vi "TestTime_PublishAndObserve_OneTopic.vi"(8 "error in (no error)":errorcluster, 11 "TestCase in":refnum<class "BenchmarkObservationRate.lvclass">) -> (0 "error out":errorcluster, 3 "TestCase out":refnum<class "BenchmarkObservationRate.lvclass">)   [LabVIEW 2020, in "BenchmarkObservationRate.lvlib" / "BenchmarkObservationRate.lvclass"]
uses:
  BenchmarkObservationRate.lvclass
  BenchmarkObservationRate.lvclass/BenchmarkObservationRate.ctl
  24bf8875-c008-4f22-9bfa-88e42476d167.vi
  Source/IModel/IModel/IModel.lvclass
  <vilib>/ActorFramework/Actor/Actor.lvclass
  Source/Mediator/Mediator/Mediator.lvclass
  <vilib>/ActorFramework/Stop Msg/Stop Msg.lvclass
  Doubles/RootModelPublishesUnthrottled/ModelPublishesIndexA.lvclass
  Doubles/ModelCountsObservations/ModelTimesNObservations.lvclass
  Source/RootModel/RootModel/RootModel.lvclass
  C:/Git/mva-core/Source/IModel/IModel/IModel.lvclass
  C:/Git/mva-core/Source/IObserver/IObserver/IObserver.lvclass
  C:/Program Files (x86)/National Instruments/LabVIEW 2020/vi.lib/ActorFramework/Actor/Actor.lvclass
  C:/Git/mva-core/Source/RootModel/RootModel/RootModel.lvclass
  C:/Git/mva-core/Test/BechmarkObservationRate/Doubles/RootModelPublishesUnthrottled/ModelPublishesIndexA.lvclass
  C:/Git/mva-core/Test/BechmarkObservationRate/Doubles/ModelCountsObservations/ModelTimesNObservations.lvclass
panel:
  out "Publish-Observe Rate [Hz]":dbl
  out "Total Time [s]":dbl
  # "About 12 kHz typical in LV 2017"
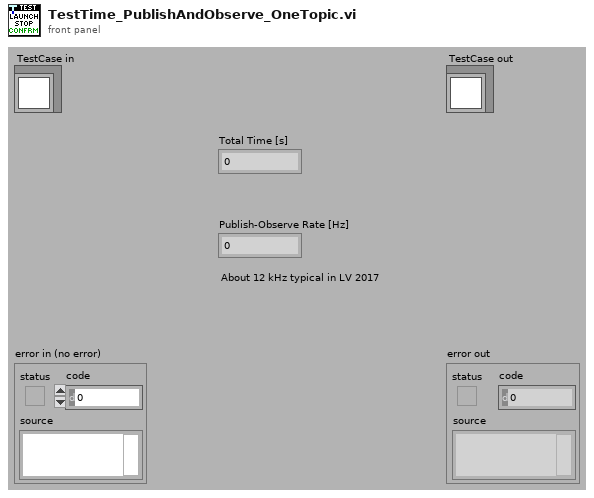
[diagram p1: front panel]
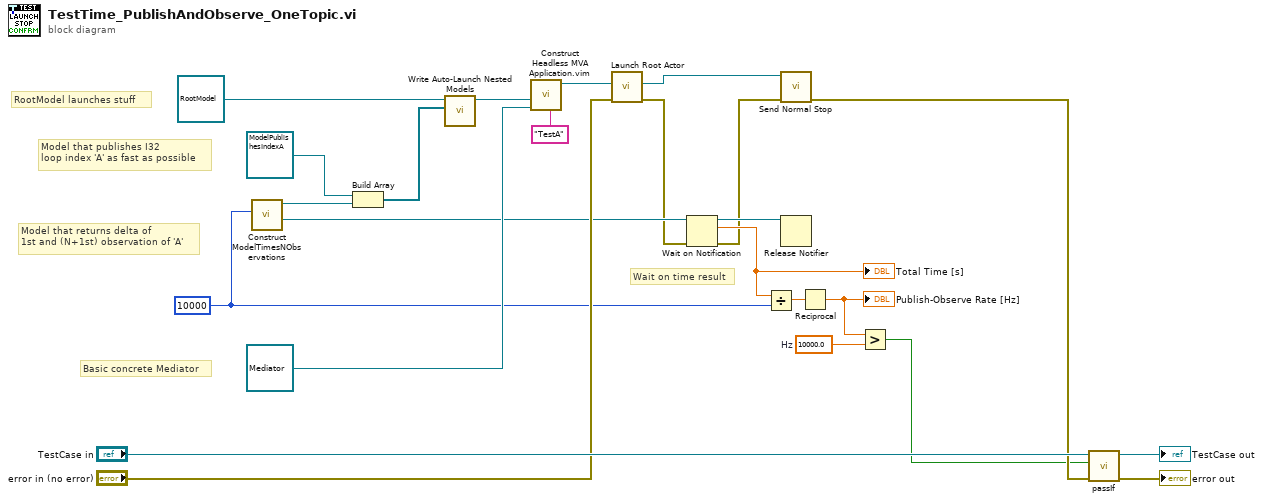
[diagram p0: block diagram]
diagram:
  w3 = 10000.0  # Hz
  w6 = 10000 ("Stop After N Observations")
  # "Wait on time result"
  # "RootModel launches stuff"
  # "Model that returns delta of\n1st and (N+1st) observation of 'A'"
  # "Model that publishes I32\nloop index 'A' as fast as possible"
  # "Basic concrete Mediator"
  n1 = call "Construct ModelTimesNObservations.vi"("Stop After N Observations"=w6) -> ("Elaped Seconds"=w13:refnum<notifier>, "ModelCountsObservations Out"=w12:refnum<class "ModelTimesNObservations.lvclass">)  [unwired: 9 in]
  n2 = Build Array(refnum<class "ModelPublishesIndexA.lvclass"> refnum ("BenchmarkObservationRate.lvlib:RootModelPublishesUnthrottled.lvclass"), w12) -> (w21:refnum<class "IModel.lvclass">[])
  n3 = call "Write Auto-Launch Nested Models.vi"("Auto-Launch Nested Models"=w21, "IModel In"=refnum<class "RootModel.lvclass"> refnum ("RootModel.lvlib:RootModel.lvclass")) -> ("IModel Out"=w20:refnum<class "RootModel.lvclass">)  [unwired: 9 in]
  n4 = call "Construct Headless MVA Application.vim"("Application Instance Alias"="TestA", "Mediator Type"=refnum<class "Mediator.lvclass"> refnum ("Mediator.lvlib:Mediator.lvclass"), "RootModel in"=w20) -> ("RootModel out"=w19:refnum<class "RootModel.lvclass">)  [unwired: 8 in]
  n5 = call <vilib>:"Launch Root Actor.vi"("error in (no error)"="error in (no error)", "Actor"=w19) -> ("error out"=w11:errorcluster, "Actor's Enqueuer"=w15:refnum<class "Message Enqueuer.lvclass">)  [unwired: 8 in]
  n6 = Wait on Notification(notifier=w13, error in (no error)=w11) -> (notifier out=w14:refnum<notifier>, notification=w7:dbl, error out=w1:errorcluster)  [unwired: 2 in, 1 out]
  "Total Time [s]" <- w7
  n7 = Divide(x=w7, y=w6) -> (x/y=w5:dbl)
  n8 = call <vilib>:"Send Normal Stop.vi"("error in (no error)"=w1, "Message Enqueuer"=w15) -> ("error out"=w10:errorcluster)  [unwired: 9 in]
  n9 = Release Notifier(notifier=w14) -> ()  [unwired: 2 in, 3 out]
  n10 = Reciprocal(x=w5) -> (1/x=w4:dbl)
  "Publish-Observe Rate [Hz]" <- w4
  n11 = Greater?(x=w4, y=w3) -> (0:w2:bool)
  n12 = call-dynamic "passIf.vi"("error in (no error)"=w10, "pass"=w2, "TestCase in"="TestCase in") -> ("error out"=→"error out":errorcluster, "TestCase out"=→"TestCase out":refnum<class "BenchmarkObservationRate.lvclass">)  [unwired: 7 in]
